vi "Core Action.vi"(8 "error in (no error)":errorcluster, 10 "SECS-II Class":refnum<class "SECS-II Class.lvclass">, 11 "25-Host Accepts Off-Line in":refnum<class "25-Host Accepts Off-Line.lvclass">) -> (0 "error out":errorcluster, 2 "SECS-II Class Out":refnum<class "SECS-II Class.lvclass">, 3 "25-Host Accepts Off-Line out":refnum<class "25-Host Accepts Off-Line.lvclass">)   [LabVIEW 2020, in "SECS Scenarios.lvlib" / "25-Host Accepts Off-Line.lvclass"]
uses:
  25-Host Accepts Off-Line.lvclass
  D:/Dropbox/SECS/SECS_GEM v1.1.0/Com/SECS Scenarios/Scenarios Class/Scenarios Class.lvclass
  SECS Communication/SECS-II Class/SECS-II Class.lvclass
  25-Host Accepts Off-Line.lvclass/25-Host Accepts Off-Line.ctl
  Write Off-Line.vi
  Scenarios Class/Scenarios Class.lvclass
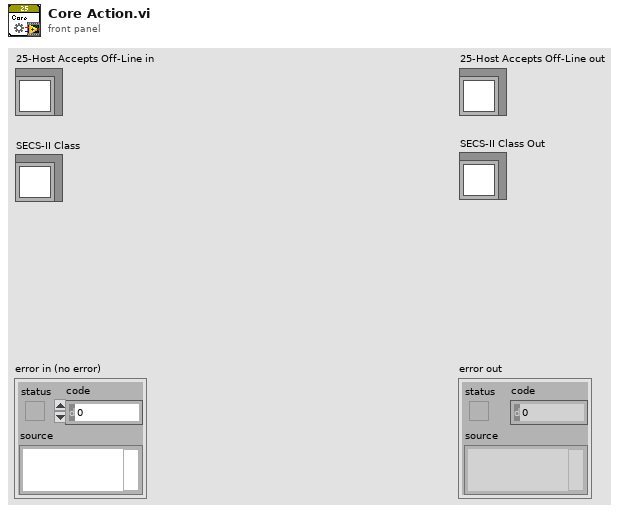
[diagram p1: front panel]
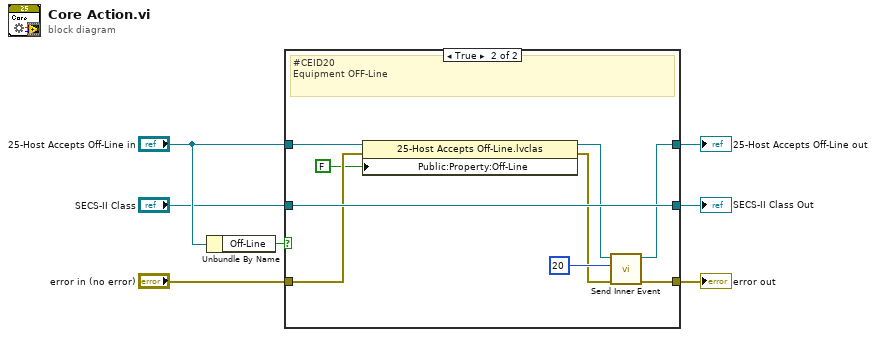
[diagram p0: block diagram]
diagram:
  n1 = Unbundle By Name("25-Host Accepts Off-Line in") -> ("Off-Line"=w7:bool)
  n2 = case shown="True" w7 {
    tunnel: "25-Host Accepts Off-Line in" -> [w9 w18]
    tunnel: "error in (no error)" -> [w10 w17]
    tunnel: [w10 w15] -> w3
    tunnel: [w9 w11] -> w4
    tunnel: "SECS-II Class" -> [w8 w19]
    tunnel: [w8 w19] -> w1
    frame False {
    }
    frame True {
      # "#CEID20\nEquipment OFF-Line"
      n3 = property class="25-Host Accepts Off-Line.lvclas"(reference=w18, error in=w17, "Public:Property:Off-Line"=FALSE ("Off-Line")) -> (reference out=w13:refnum<class "25-Host Accepts Off-Line.lvclass">, error out=w12:errorcluster)
      n4 = call "Send Inner Event.vi"("error in (no error)"=w12, "CEID"=u32 20, "Scenarios Class in"=w13) -> ("error out"=w15:errorcluster, "Scenarios Class out"=w11:refnum<class "25-Host Accepts Off-Line.lvclass">)  [unwired: 7 in]
    }
  }
  "error out" <- w3
  "25-Host Accepts Off-Line out" <- w4
  "SECS-II Class Out" <- w1
